vi "Request Data JSON.vi"(8 "error in (no error)":errorcluster, 11 "GetInputVolume in":refnum<class "GetInputVolume.lvclass">) -> (0 "error out":errorcluster, 2 "Request Data JSON":string, 3 "GetInputVolume out":refnum<class "GetInputVolume.lvclass">)   [LabVIEW 2020, in "obs-websocket.lvlib" / "GetInputVolume.lvclass"]
uses:
  GetInputVolume.lvclass
  GetInputVolume.lvclass/GetInputVolume.ctl
  982caa60-3be5-414e-94b8-d7d2ee2e07af.vi
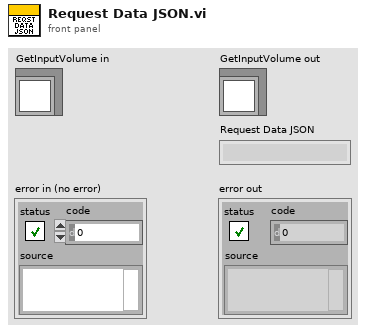
[diagram p1: front panel]
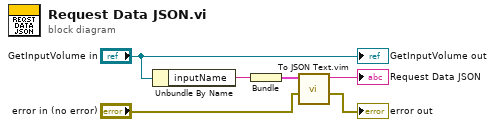
[diagram p0: block diagram]
diagram:
  n1 = Unbundle By Name("GetInputVolume in") -> ("inputName"=w5:string)
  n2 = Bundle("inputName"=w5) -> (w4:cluster{"inputName":string})  [unwired: 1 in]
  n3 = call "To JSON Text.vim"("error in (no error)"="error in (no error)", "Anything"=w4) -> ("error out"=→"error out":errorcluster, "<JSON>"=→"Request Data JSON":string)  [unwired: 8 in]
  "GetInputVolume out" <- "GetInputVolume in"
